vi "Parse.vi"(8 "Error In":errorcluster, 11 "object in":refnum<class "2021_15.lvclass">) -> (0 "Error Out":errorcluster, 3 "object out":refnum<class "2021_15.lvclass">)   [LabVIEW 2020, in "2021_15.lvclass"]
uses:
  2021_15.lvclass
  2021_15.lvclass/2021_15.ctl
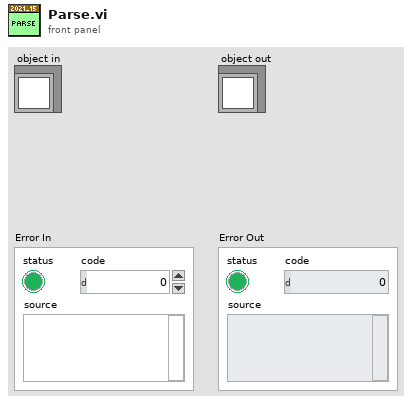
[diagram p1: front panel]
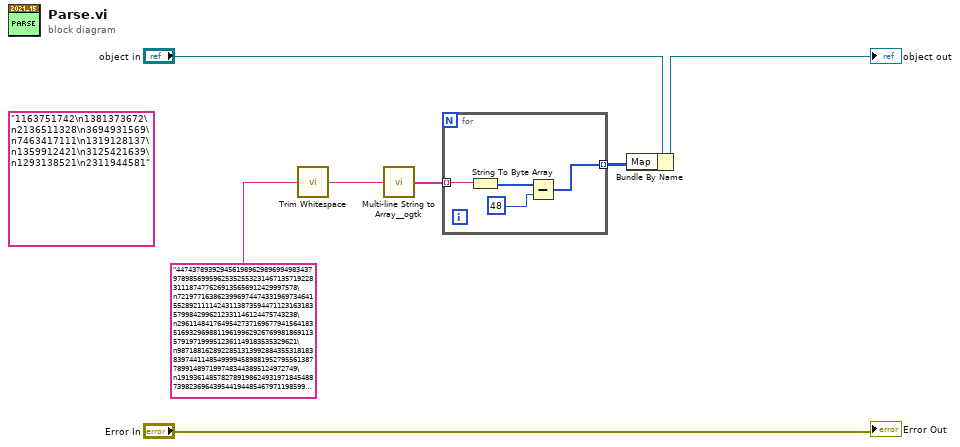
[diagram p0: block diagram]
diagram:
  (unwired) "1163751742\n1381373672\n2136511328\n3694931569\n7463417111\n1319128137\n1359912421\n3125421639\n1293138521\n2311944581"
  n1 = call <vilib>:"Trim Whitespace.vi"("string"="4474378939294561989629896994983437978985699596253525532314671357192283111874776269135656912429997578\n7219771638623996974474331969734641552892111142431138735944711231631835799842996212331146124475743238\n2961148417649542737169677941564183516932969881196199629267699818691135791971999512361149183535329621\n9871881628922851313992884355318183839744114854999945898819527955613877899148971997483443895124972749\n1919361485782789198624931971845488739823696439544194485467971198599719115839184879611199597989117999\n17626684653189871686799282735487523264939254458987125749992718721494114139545671491283213567137...") -> ("trimmed string"=w2:string)  [unwired: 1 in]
  n2 = call <userlib>:"Multi-line String to Array__ogtk.vi"("string"=w2) -> ("lines"=w3:string[])
  n3 = for {
    tunnel: [w8] -> w4 mode=indexing
    tunnel: w3 -> [w11] mode=indexing
    n4 = String To Byte Array(string=w11) -> (unsigned byte array=w10:u8[])
    n5 = Subtract(x=w10, y=u8 48) -> (x-y=w8:u8[])
  }
  n6 = Bundle By Name(cluster="object in", "Map"=w4) -> (→"object out":refnum<class "2021_15.lvclass">)
  "Error Out" <- "Error In"
